vi "计算.vi"(8 "error in (no error)":errorcluster caption="错误输入（无错误）", 11 "运算类 输入":refnum<class "运算类.lvclass"> caption="DNL_LabVIEW Object in") -> (0 "error out":errorcluster caption="错误输出", 2 "结果":dbl, 3 "运算类 输出":refnum<class "运算类.lvclass"> caption="DNL_LabVIEW Object out")   [LabVIEW 2013, in "运算类.lvclass"]
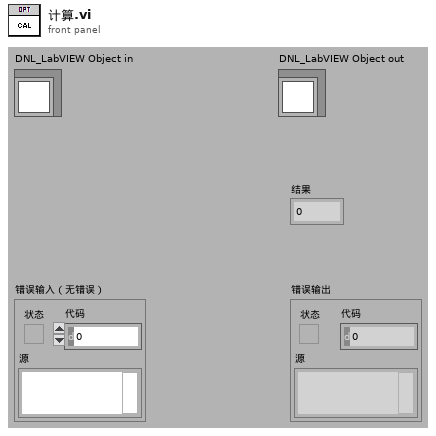
[diagram p1: front panel]
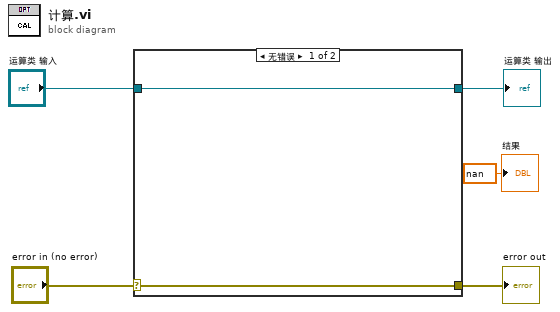
[diagram p0: block diagram]
diagram:
  n1 = case shown="无错误" "error in (no error)" {
    selector: "error in (no error)" -> [w6 w9]
    tunnel: [w6 w9] -> w4
    tunnel: [w7 w8] -> w2
    tunnel: "运算类 输入" -> [w7 w8]
    frame No Error {
    }
    frame Error {
    }
  }
  "error out" <- w4
  "运算类 输出" <- w2
  "结果" <- nan ("结果")
